vi "Create Oneof Message Converters (Rich to Flat).vi"(8 "error in (no error)":errorcluster, 10 "message parameters":T1[](array[typedef]), 11 "library in":refnum<vi>) -> (0 "error out":errorcluster, 3 "library out":refnum<vi>)   [LabVIEW 2019, in "gRPC Template Creation Utility.lvlib"]
uses:
  gRPC Template Creation Utility.lvlib
  OneOf Constants/OneOfConstantsEnum.ctl
  TypeDefs/Message Metadata (Scripting).ctl
  TypeDefs/Message Element Type.ctl
  TypeDefs/Message Element Metadata (Scripting).ctl
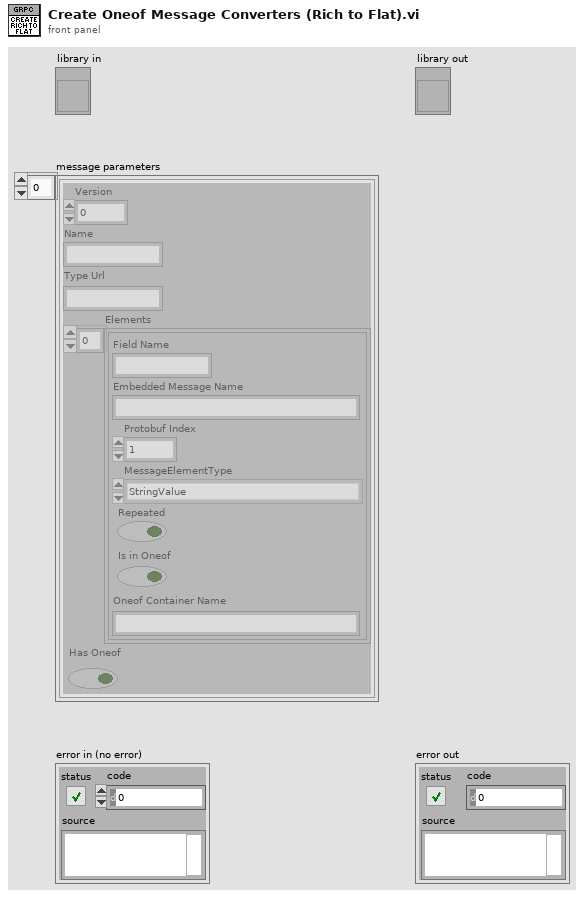
[diagram p1: front panel]
types:
  T1 = typedef "gRPC Template Creation Utility.lvlib/Message Metadata (Scripting).ctl" = cluster{"Version":i32, "Name":string, "Type Url":string, "Elements":T2[], "Has Oneof":bool}
  T2 = typedef "gRPC Template Creation Utility.lvlib/Message Element Metadata (Scripting).ctl" = cluster{"Field Name":string, "Embedded Message Name":string, "Protobuf Index":i32, "MessageElementType":T3, "Repeated":bool, "Is in Oneof":bool, "Oneof Container Name":string}
  T3 = typedef "gRPC Template Creation Utility.lvlib/Message Element Type.ctl" = enum32{"Int32Value", "FloatValue", "DoubleValue", "BoolValue", "StringValue", "MessageValue", "Int64Value", "UInt32Value", "UInt64Value", "EnumValue", "Bytes", "Fixed64", "Fixed32", "SFixed64", "SFixed32", "SInt64", "SInt32"}
  T4 = typedef "gRPC Template Creation Utility.lvlib/OneOfConstantsEnum.ctl" = enum16{"FlatToRichVIPrefix", "RichToFlatVIPrefix", "FlatTypeDefSuffix"}
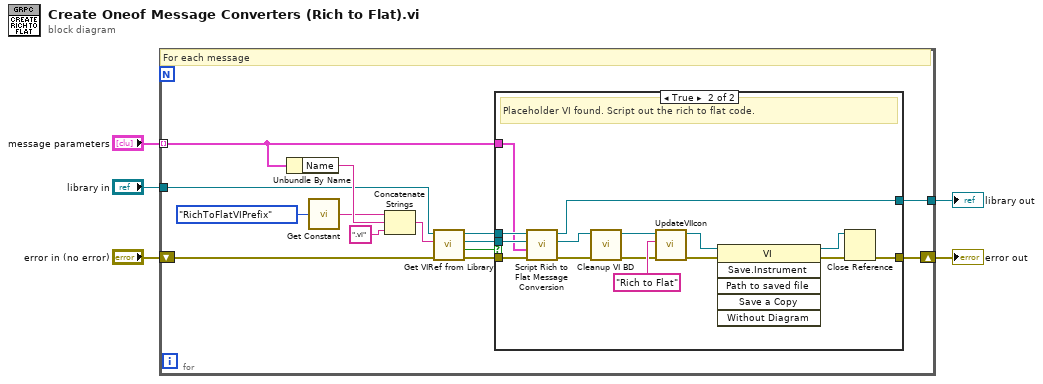
[diagram p0: block diagram]
diagram:
  n1 = for {
    tunnel: "message parameters" -> [w17] mode=indexing
    shift-right: [w18] -> w3
    shift-left: "error in (no error)" -> [w6]
    tunnel: "library in" -> [w7]
    tunnel: [w19] -> w5
    # "For each message"
    n2 = Unbundle By Name(w17) -> ("Name"=w10:string)
    n3 = call "Get Constant.vi"("Selection"=OneOfConstantsEnum."RichToFlatVIPrefix") -> ("String"=w8:string)
    n4 = Concatenate Strings(w8, w10, ".vi" ("string")) -> (w15:string)
    n5 = call "Get VIRef from Library.vi"("error in (no error)"=w6, "item name"=w15, "library in"=w7) -> ("error out"=w11:errorcluster, "found"=w13:bool, "vi"=w14:refnum<vi>, "library out"=w12:refnum<vi>)  [unwired: 5 in]
    n6 = case shown="True" w13 {
      tunnel: w11 -> [w21 w36]
      tunnel: [w20 w35] -> w19
      tunnel: [w21 w23] -> w18
      tunnel: w14 -> [_ w33]
      tunnel: w12 -> [w20 w34]
      tunnel: w17 -> [_ w32]
      frame False {
      }
      frame True {
        # "Placeholder VI found. Script out the rich to flat code."
        n7 = call "Script Rich to Flat Message Conversion.vi"("error in (no error)"=w36, "message metadata"=w32, "vi in"=w33, "library in"=w34) -> ("error out"=w31:errorcluster, "vi out"=w30:refnum<vi>, "library out"=w35:refnum<vi>)  [unwired: 5 in]
        n8 = call "Cleanup VI BD.vi"("error in (no error)"=w31, "VI in"=w30) -> ("error out"=w28:errorcluster, "VI out"=w27:refnum<vi>)  [unwired: 8 in]
        n9 = call "UpdateVIIcon.vi"("error in (no error)"=w28, "Method Name"="Rich to Flat", "VI in"=w27) -> ("error out"=w25:errorcluster, "VI out"=w26:refnum<vi>)  [unwired: 7 in]
        n10 = invoke class="VI" method="Save.Instrument"(reference=w26, error in=w25) -> (reference out=w22:refnum<vi>, error out=w24:errorcluster)  [unwired: 4 in, 4 out]
        n11 = Close Reference(reference=w22, error in (no error)=w24) -> (error out=w23:errorcluster)
      }
    }
  }
  "library out" <- w5
  "error out" <- w3
